vi "Write aborted.vi"(8 "error in (no error)":errorcluster, 10 "aborted":bool, 11 "S4ACS_GUI in":refnum<class "S4ACS_GUI.lvclass">) -> (0 "error out":errorcluster, 3 "S4ACS_GUI out":refnum<class "S4ACS_GUI.lvclass">)   [LabVIEW 2018, in "S4ACS_GUI.lvclass"]
uses:
  S4ACS_GUI.lvclass
  S4ACS_GUI.lvclass/S4ACS_GUI.ctl
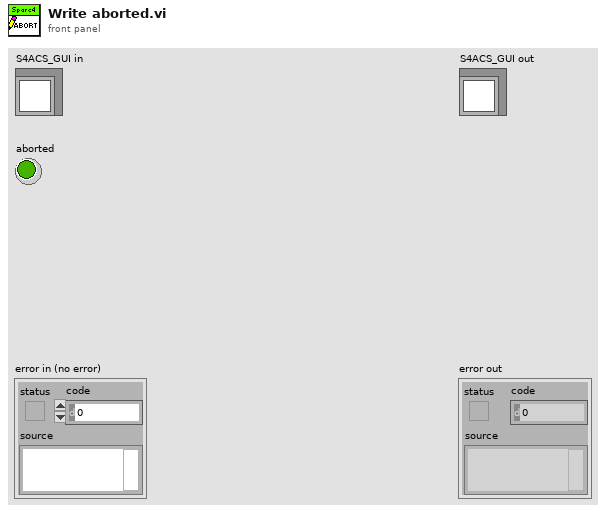
[diagram p1: front panel]
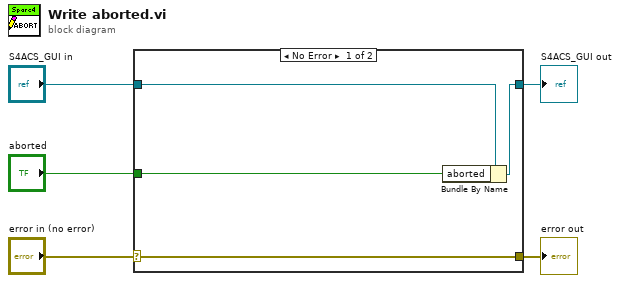
[diagram p0: block diagram]
diagram:
  n1 = case shown="No Error" "error in (no error)" {
    selector: "error in (no error)" -> [w9 w10]
    tunnel: [w9 w10] -> w4
    tunnel: [w7 w11] -> w2
    tunnel: "S4ACS_GUI in" -> [w8 w11]
    tunnel: "aborted" -> [w6 _]
    frame No Error {
      n2 = Bundle By Name(cluster=w8, "aborted"=w6) -> (w7:refnum<class "S4ACS_GUI.lvclass">)
    }
    frame Error {
    }
  }
  "error out" <- w4
  "S4ACS_GUI out" <- w2
